vi "bon format designation.vi"(1 "Chaîne IN":string="       417mA       14.4ohm       ") -> (0 "Chaîne OUT":string="417mA 14.4ohm")   [LabVIEW 2020]
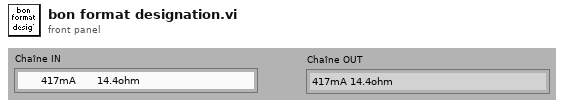
[diagram p1: front panel]
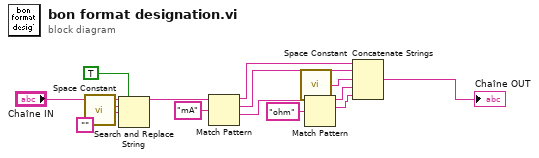
[diagram p0: block diagram]
diagram:
  n1 = call <vilib>:"Space Constant.vi"() -> ("String"=w12:string)
  n2 = Search and Replace String(replace all?=TRUE ("tout remplacer ? (F)"), input string="Chaîne IN", search string=w12, replace string="" ("chaîne recherchée")) -> (result string=w10:string)  [unwired: 4 in, 3 out]
  n3 = Match Pattern(string=w10, regular expression="mA" ("expression régulière")) -> (before substring=w4:string, match substring=w3:string, after substring=w8:string)  [unwired: 1 in, 1 out]
  n4 = call <vilib>:"Space Constant.vi"() -> ("String"=w5:string)
  n5 = Match Pattern(string=w8, regular expression="ohm" ("expression régulière")) -> (before substring=w6:string, match substring=w1:string)  [unwired: 1 in, 2 out]
  n6 = Concatenate Strings(w4, w3, w5, w6, w1) -> (→"Chaîne OUT":string)
